vi "Init Godot.vi"(8 "error in (no error)":errorcluster, 11 "FormulaLV App in":refnum<class "FormulaG App.lvclass">) -> (0 "error out":errorcluster, 3 "FormulaLV App out":refnum<class "FormulaG App.lvclass">)   [LabVIEW 2020, in "FormulaG.lvlib" / "FormulaG App.lvclass"]
uses:
  FormulaG App.lvclass
  FormulaG App.lvclass/FormulaG App.ctl
  <vilib>/IlluminatedG/IG GodotServer/GodotLV/GodotServer/GodotServer.lvclass
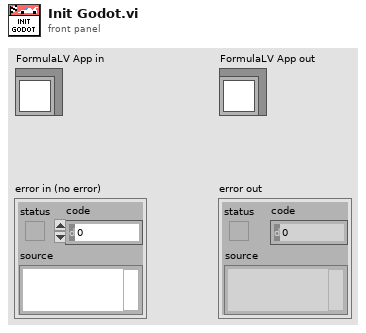
[diagram p1: front panel]
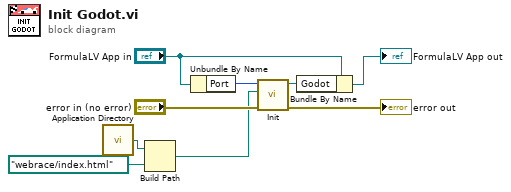
[diagram p0: block diagram]
diagram:
  n1 = call <vilib>:"Application Directory.vi"() -> ("Application Directory"=w8:path)
  n2 = Build Path(base path=w8, name or relative path=path "webrace/index.html") -> (appended path=w5:path)
  n3 = Unbundle By Name("FormulaLV App in") -> ("Port"=w1:u16)
  n4 = call <vilib>:"Init.vi"("error in (no error)"="error in (no error)", "Godot Export HTML"=w5, "Port (10027)"=w1) -> ("error out"=→"error out":errorcluster, "GodotServer out"=w4:refnum<class "GodotServer.lvclass">)  [unwired: 7 in]
  n5 = Bundle By Name(cluster="FormulaLV App in", "Godot"=w4) -> (→"FormulaLV App out":refnum<class "FormulaG App.lvclass">)
